vi "5785_3200MHz_multi emitter.vi"() -> ()   [LabVIEW 2021]
uses:
  <instrlib>/_niInstr/Streaming/v1/Common/Stream State.ctl
  <vilib>/Platform/TimedLoop/XDataNode/timing_clust.ctl
  <vilib>/Platform/TimedLoop/XDataNode/nitl_modes.ctl
  <vilib>/Platform/TimedLoop/XDataNode/wakeup.ctl
  <instrlib>/FlexRIO/API/FPGA/v1/Types/Start Trigger IO Resources.ctl
  <instrlib>/_niInstr/DSP/v1/Shared/Public/IQ Data.ctl
  <vilib>/rvi/Emulation/niFpgaSctlEmulationGetInTimedLoop.vi
  <vilib>/rvi/Emulation/niFpgaEmulationReportErrorSimple.vi
  <vilib>/rvi/Emulation/niFpgaGetClockAttributes.vi
  <vilib>/rvi/Emulation/niFpgaCriticalErrorInLSC.vi
  7192f61d-e408-4cca-baff-cb10c33219c0.vi
  <vilib>/rvi/interface/RandomDataEmulation/nirviRandomDataMultiElementFPGAFIFO.vi
  <instcachedir>/0/nirviRandomDataMultiElementFPGAFIFO_3E9965BA1FAD4E7B8DABA31768A09B1F.lvgen/nirviRandomDataMultiElementFPGAFIFO_3E9965BA1FAD4E7B8DABA31768A09B1F_000.vi
  <vilib>/rvi/interface/RandomDataEmulation/niFpgaRandomDataHandleErrors.vi
  <vilib>/rvi/eio/common/nirviEmuTemplateMethod_errors.vi
  <vilib>/Platform/TimedLoop/XDataNode/XDataNode.xnode
  <vilib>/rvi/DataTransferAndStorage/Container/XNode/niFpgaContainer.xnode
  <vilib>/rvi/interface/RandomDataEmulation/nirviRandomDataFpgaMultiElementTemplate.vi
  <vilib>/eio/EIONode/EIONode.xnode
  <vilib>/Platform/TimedLoop/XDataNode/XDNodeRunTimeDep.lvlib
  <instrlib>/_niInstr/Streaming/v1/FPGA/niInstr Streaming v1 FPGA.lvlib
  <instrlib>/FlexRIO/API/FPGA/v1/FlexRIO API FPGA v1.lvlib
  <instrlib>/FlexRIO/API/FPGA/v1/IO/NI5785/FlexRIO 5785 FPGA v1.lvlib
  <instrlib>/_niInstr/DSP/v1/Shared/niInstr DSP v1 Shared.lvlib
  <instrlib>/_niInstr/Basic Elements/v1/FPGA/niInstr Basic Elements v1 FPGA.lvlib
  <instrlib>/_niInstr/Streaming/v1/Common/niInstr Streaming v1 Common.lvlib
panel:
  out "pulse TX status":T1
  in  "reset system clock":bool
  in  "User-defined Start Trigger - AO":bool
  in  "flexrio.trigger.start.cfg 1":u16
  out "IO Socket\\AO Ready For Input":bool
  in  "stream.request state 1":T2
  in  "stream.num samples 1":u64
  out "stream.metadata 1":u64
  out "stream.samples transferred 1":u64
  out "stream.state 1":T2
  out "flexrio.module.io ready 0":bool
  out "flexrio.module.io error 0":i32
  out "flexrio.module.data valid 0":bool
  # "Data Path Configuration"
  # "AI Trigger Configuration"
  # "AI Stream Configuration"
  # "AO Stream Configuration"
  # "Module Status"
  # "AO Buffer Configuration"
  # "Device Utilization\n---------------------------\nTotal Slices: 62.6% (18977 out of 30300)\nSlice Registers: 23.8% (115206 out of 484800)\nSlice LUTs: 38.2% (92532 out of 242400)\nBlock RAMs: 56.8% (341 out of 600)\nDSP48s: 0.3% (6 out of 1920)\n\nNote: Utilization numbers are for the KU040. Exact values will vary for the KU060 and KU035."
  # "User-defined Controls"
  # "AO Trigger Configuration"
  # "Utilization numbers are for the KU060."
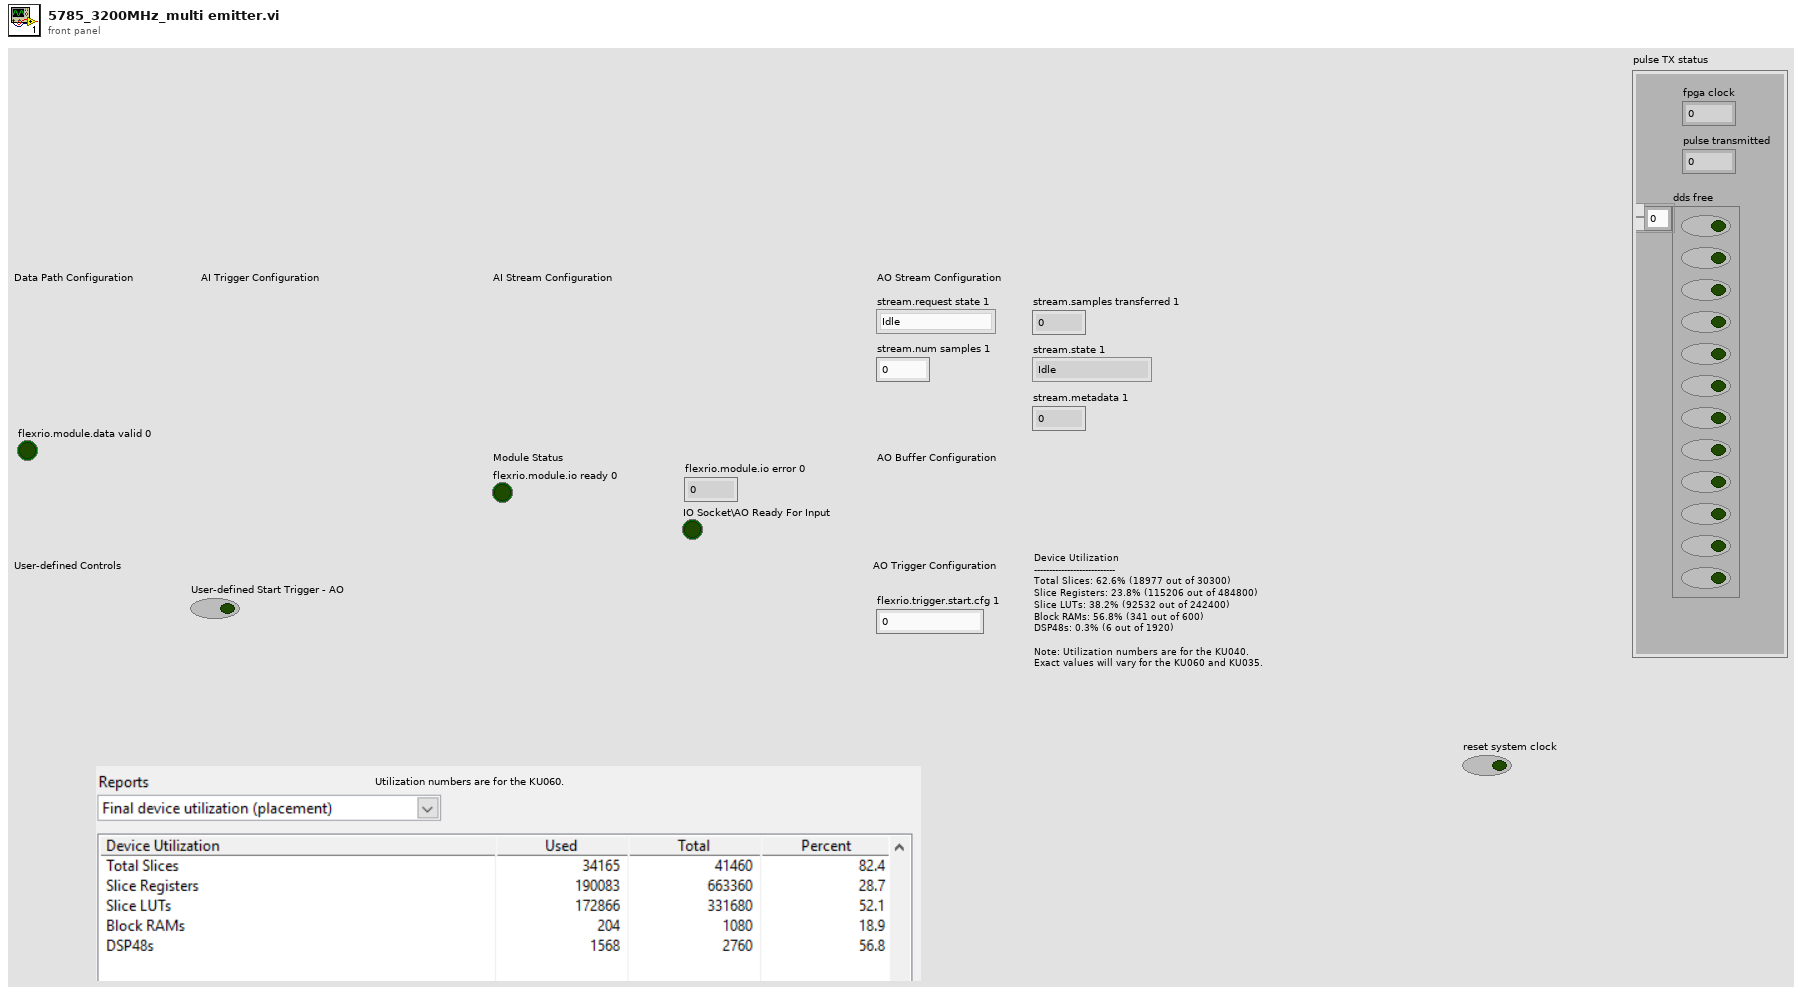
[diagram p1: front panel]
types:
  T1 = cluster{"fpga clock":u64, "pulse transmitted":u32, "dds free":bool[]}
  T2 = typedef "niInstr Streaming v1 Common.lvlib/Stream State.ctl" = enum8{"Idle", "Finite Transfer", "Continuous", "Done", "Error", "Not Ready", "Cancel"}
  T3 = typedef "XDNodeRunTimeDep.lvlib/timing_clust.ctl" = cluster{"Expected End [f-1]":u64, "Actual End [f-1]":u64, "Finished Late? [f-1]":bool, "Expected End [i-1]":u64, "Actual End [i-1]":u64, "Finished Late? [i-1]":bool, "Expected Start [i]":u64, "Actual Start [i]":u64, "Expected Start [f]":u64, "Actual Start [f]":u64, "Source Name":string, "Structure Name":string, "Period":i64, "Deadline":i64, "Offset":i64, "Start":i64, "Priority":i32, "Timeout":i32, "Mode":T4, "Wakeup Reason":T5, "Error":errorcluster, "Source Type":string, "Secondary Source Type":string, "Global End Time":u64, "Global Start Time":u64, "Frame Duration":u64, "Iteration Duration":u64, "Assigned CPU":i32, "I/O Scan Engine Mode":u32}
  T4 = typedef "XDNodeRunTimeDep.lvlib/nitl_modes.ctl" = enum32{"No Change", "Process missed periods, maintain original phase", "Discard missed periods, maintain original phase", "Process missed periods, ignore original phase", "Discard missed periods, ignore original phase"}
  T5 = typedef "XDNodeRunTimeDep.lvlib/wakeup.ctl" = enum32{"Normal", "Aborted", "Asynchronous wakeup", "Timing source error", "Timed loop error", "Timeout"}
  T6 = typedef "niInstr DSP v1 Shared.lvlib/IQ Data.ctl" = cluster{"I":fxp<+/-,18,1>, "Q":fxp<+/-,18,1>, "overflow":bool}
  T7 = typedef "FlexRIO API FPGA v1.lvlib/Start Trigger IO Resources.ctl" = cluster{"start trigger":refnum<k21>, "started event":refnum<k21>, "start trigger for export":refnum<k21>, "start trigger for tclk":refnum<k21>}
  T8 = typedef "FlexRIO API FPGA v1.lvlib/Start Trigger Control.ctl" = cluster{"arm start":bool, "done":bool}
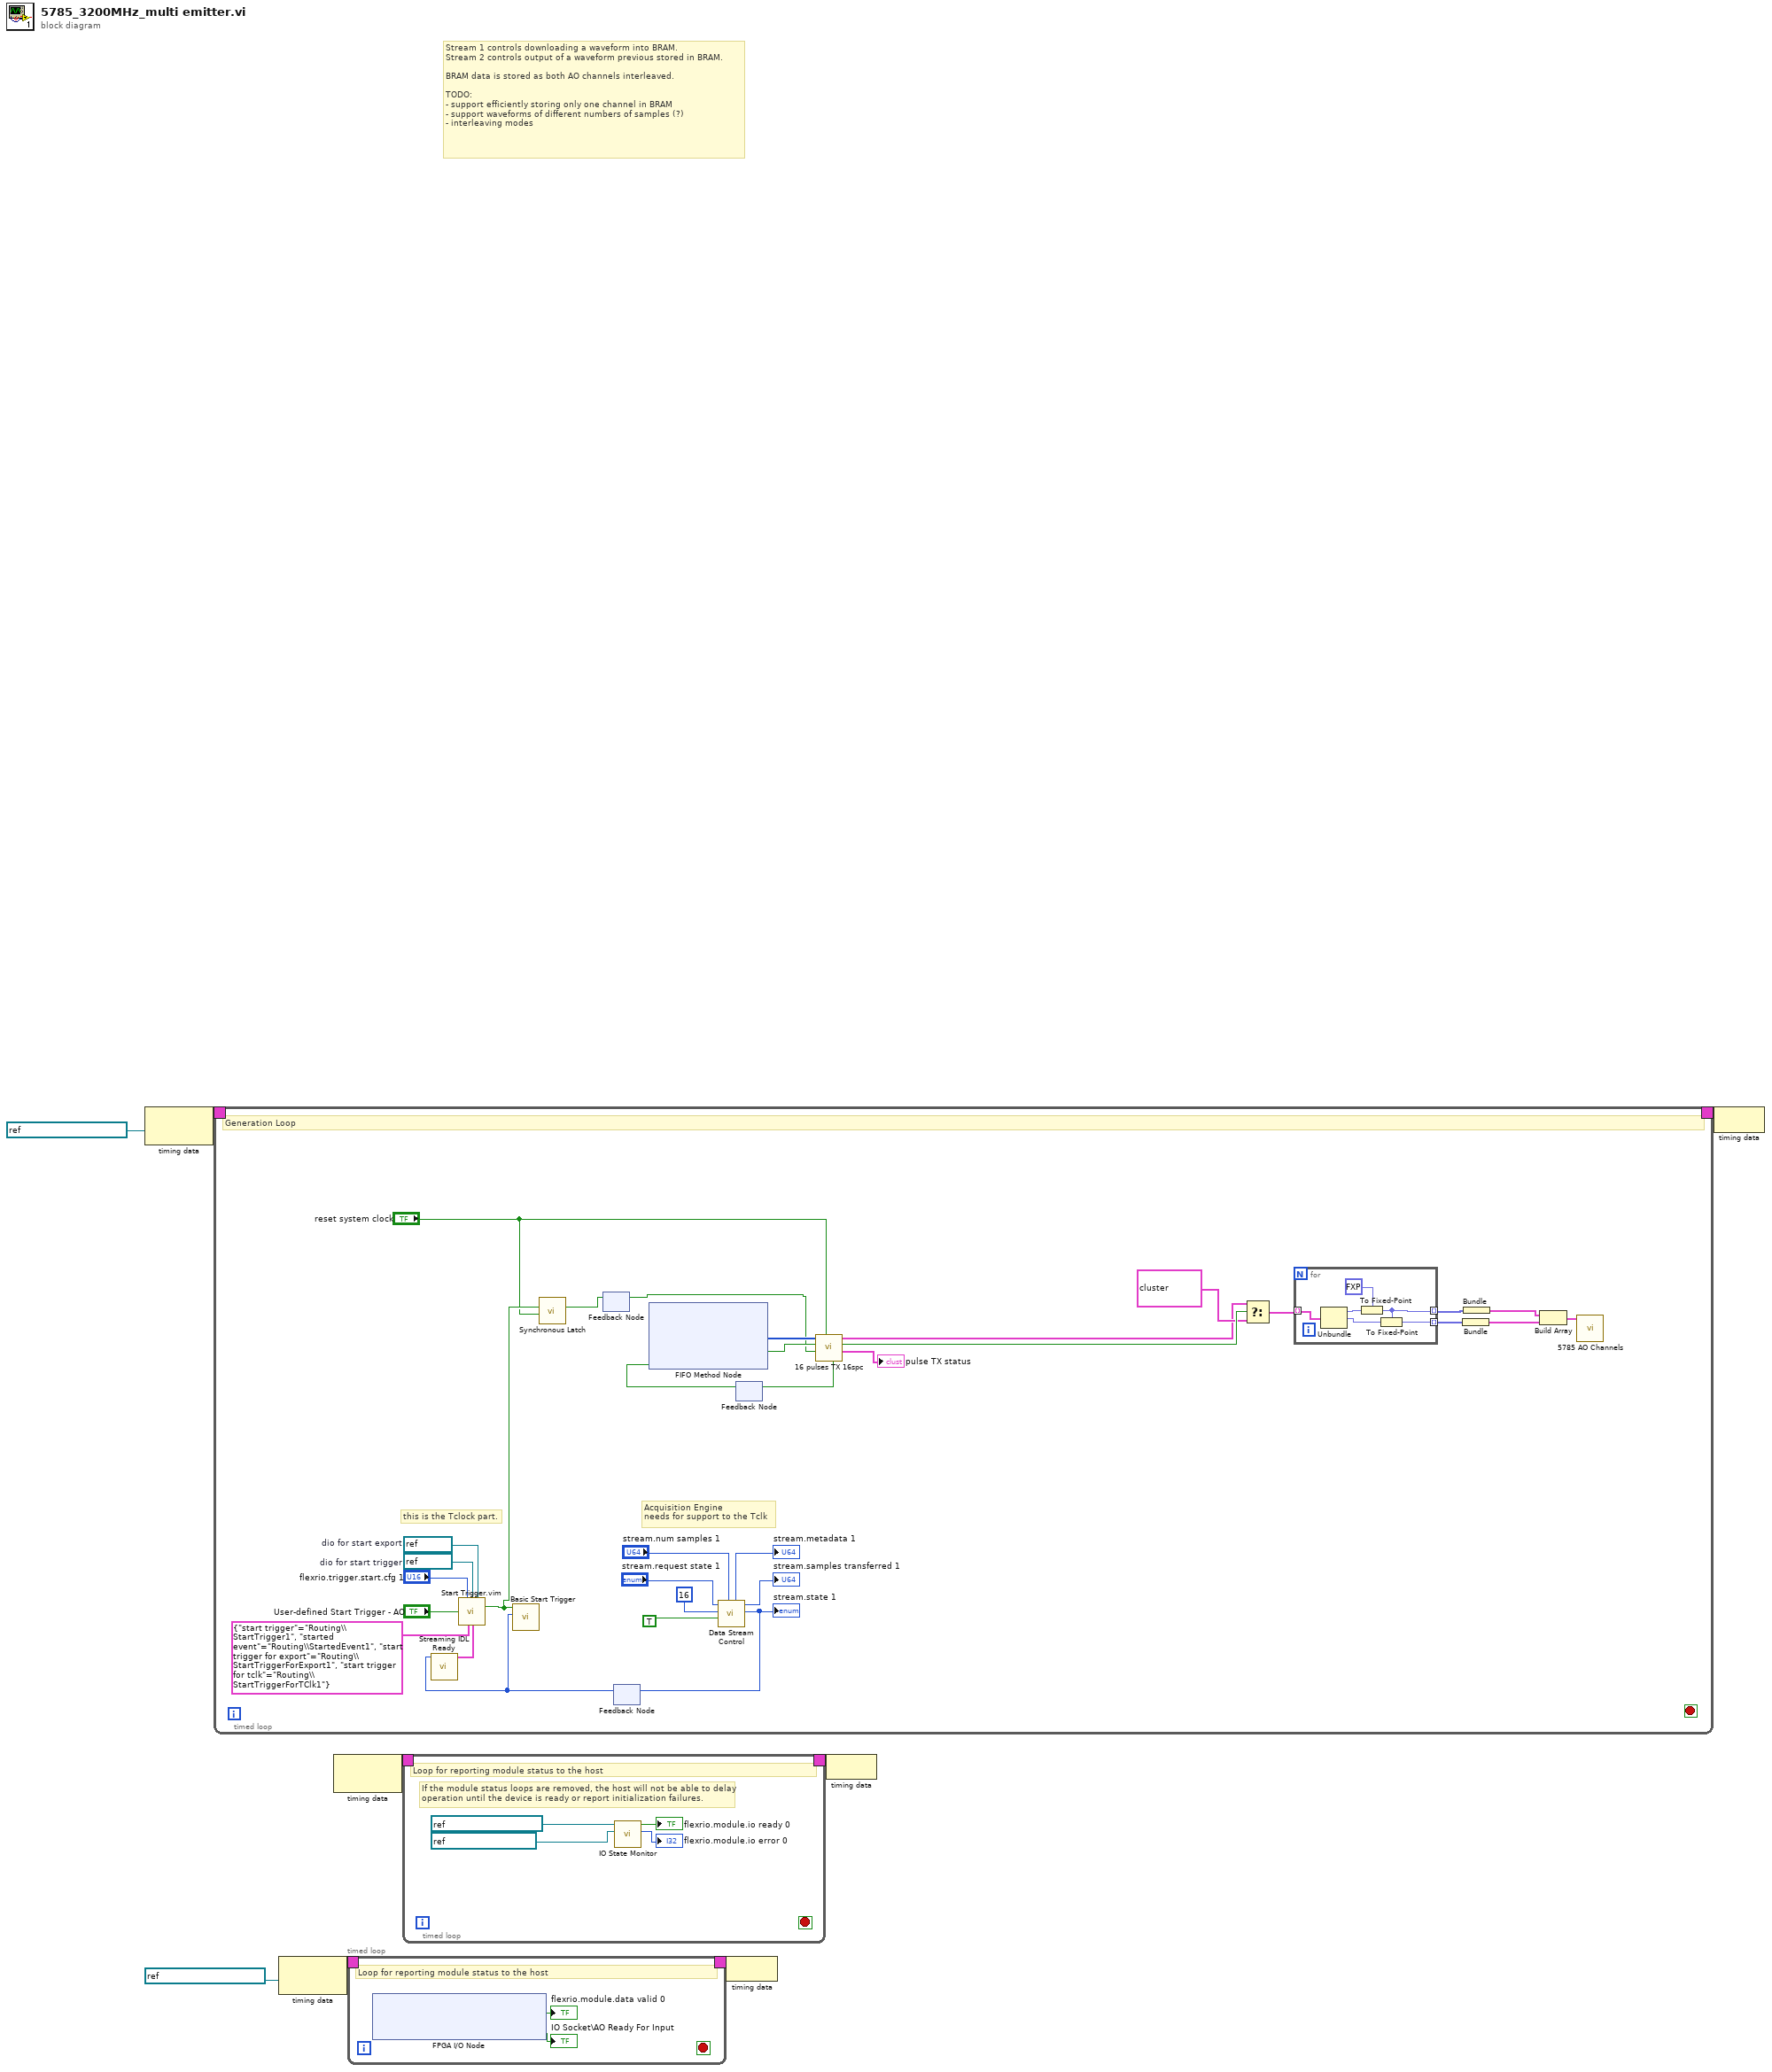
[diagram p0: block diagram]
diagram:
  # "Stream 1 controls downloading a waveform into BRAM.\nStream 2 controls output of a waveform previous stored in BRAM.\n\nBRAM data is stored as both AO channels interleaved.\n\nTODO:\n- support efficiently storing only one channel in BRAM\n- support waveforms of different numbers of samples (?)\n- interleaving modes"
  n1 = node-c288(refnum<k21> "IO Socket\\Data Clock" ("Source Name")) -> (w8:T3)
  n2 = timed-loop {
    timing: w8 -> [_]
    timing-out: [_] -> w7
    stop <- _ stop-if-true
    w30 = refnum<k21> "DIO 2"  # dio for start trigger
    w29 = refnum<k21> "DIO 3"  # dio for start export
    # "Acquisition Engine\nneeds for support to the Tclk"
    # "this is the Tclock part."
    # "Generation Loop"
    n3 = feedback #1() -> (w9:bool)  [unwired: 1 in]
    n4 = feedback #2() -> (w27:T2)  [unwired: 1 in]
    n5 = call <instrlib>:"Streaming IDL Ready.vi"("stream.state"=w27) -> ("start trigger control"=w31:T8)  [unwired: 10 in]
    n6 = call "Start Trigger.vim"("flexrio.trigger.start.cfg 0"="flexrio.trigger.start.cfg 1", "dio start"=w30, "dio for start export"=w29, "user-defined start trigger"="User-defined Start Trigger - AO", "trigger io resources"=T7 {"start trigger"="Routing\\StartTrigger1", "started event"="Routing\\StartedEvent1", "start trigger for export"="Routing\\StartTriggerForExport1", "start trigger for tclk"="Routing\\StartTriggerForTClk1"}, "start trigger control"=w31) -> ("conditioned start trigger"=w12:bool)  [unwired: 7 in, 2 out]
    n7 = call <instrlib>:"Basic Start Trigger.vi"("stream.state"=w27, "start trigger"=w12) -> ()  [unwired: 9 in, 1 out]
    n8 = call <instrlib>:"Synchronous Latch.vi"("clear"="reset system clock", "set"=w12) -> ("out"=w10:bool)  [unwired: 9 in]
    n9 = feedback-in #1(w10) -> ()
    n10 = call <instrlib>:"Data Stream Control.vi"("stream.num samples 0"="stream.num samples 1", "data valid"=TRUE, "element count"=u16 16, "stream.request state 0"="stream.request state 1") -> ("stream.state 0"=w33:T2, "stream.samples transferred 0"=→"stream.samples transferred 1":u64, "stream.metadata 0"=→"stream.metadata 1":u64)  [unwired: 3 in, 2 out]
    "stream.state 1" <- w33
    n11 = feedback-in #2(w33) -> ()
    n12 = feedback #3() -> (w24:bool)  [unwired: 1 in]
    n13 = xnode ("FIFO Method Node")("Ready for Output"=w24) -> ("Element"=w23:u64[], "Output Valid"=w22:bool)  [unwired: 1 in, 1 out]
    n14 = call "16 pulses TX 16spc.vi"("reset system clock"="reset system clock", "IQ_run"=w9, "PDW input Valid"=w22, "array PDW"=w23) -> ("pulse TX status"=→"pulse TX status":T1, "output valid"=w20:bool, "IQ out"=w18:T6[], "ready for input"=w25:bool)  [unwired: 4 in]
    n15 = feedback-in #3(w25) -> ()
    n16 = Select(t=w18, s=w20, f=T6[] [{"I"=0.0, "Q"=0.0, "overflow"=FALSE}, {"I"=0.0, "Q"=0.0, "overflow"=FALSE}, {"I"=0.0, "Q"=0.0, "overflow"=FALSE}, {"I"=0.0, "Q"=0.0, "overflow"=FALSE}, {"I"=0.0, "Q"=0.0, "overflow"=FALSE}, {"I"=0.0, "Q"=0.0, "overflow"=FALSE}, {"I"=0.0, "Q"=0.0, "overflow"=FALSE}, {"I"=0.0, "Q"=0.0, "overflow"=FALSE}, {"I"=0.0, "Q"=0.0, "overflow"=FALSE}, {"I"=0.0, "Q"=0.0, "overflow"=FALSE}, {"I"=0.0, "Q"=0.0, "overflow"=FALSE}, {"I"=0.0, "Q"=0.0, "overflow"=FALSE}, {"I"=0.0, "Q"=0.0, "overflow"=FALSE}, {"I"=0.0, "Q"=0.0, "overflow"=FALSE}, {"I"=0.0, "Q"=0.0, "overflow"=FALSE}, {"I"=0.0, "Q"=0.0, "overflow"=FALSE}]) -> (s? t:f=w17:T6[])
    n17 = for {
      tunnel: w17 -> [w46] mode=indexing
      tunnel: [w42] -> w21 mode=indexing
      tunnel: [w41] -> w16 mode=indexing
      n18 = Unbundle(w46) -> ("I"=w45:fxp<+/-,18,1>, "Q"=w43:fxp<+/-,18,1>)  [unwired: 1 out]
      n19 = To Fixed-Point(fixed-point type=fxp<+/-,12,1> 0.0 ("element"), number=w45) -> (fixed-point=w42:fxp<+/-,12,1>)
      n20 = To Fixed-Point(fixed-point type=w42, number=w43) -> (fixed-point=w41:fxp<+/-,12,1>)
    }
    n21 = Bundle(w16) -> (w14:cluster{fxp<+/-,12,1>[]})  [unwired: 1 in]
    n22 = Bundle(w21) -> (w15:cluster{fxp<+/-,12,1>[]})  [unwired: 1 in]
    n23 = Build Array(w15, w14) -> (w38:cluster{fxp<+/-,12,1>[]}[])
    n24 = call <instrlib>:"5785 AO Channels.vi"("all channels"=w38) -> ()  [unwired: 15 in]
  }
  n25 = node-c288(refnum<k21> "IO Socket\\Data Clock" ("Source Name")) -> (w3:T3)
  n26 = node-c288() -> (w5:T3)  [unwired: 1 in]
  n27 = timed-loop {
    timing: w3 -> [_]
    timing-out: [_] -> w2
    stop <- _ stop-if-true
    # "Loop for reporting module status to the host"
    n28 = xnode "FPGA I/O Node"() -> ("IO Socket\\AI Data Valid"=→"flexrio.module.data valid 0":bool, "IO Socket\\AO Ready For Input"=→"IO Socket\\AO Ready For Input":bool)  [unwired: 2 in, 2 out]
  }
  n29 = timed-loop {
    timing: w5 -> [_]
    timing-out: [_] -> w4
    stop <- _ stop-if-true
    # "If the module status loops are removed, the host will not be able to delay operation until the device is ready or report initialization failures."
    # "Loop for reporting module status to the host"
    n30 = call <instrlib>:"IO State Monitor.vi"("io error resource"=refnum<k21> "IO Socket\\IO Error" ("FPGA I/O In"), "io ready resource"=refnum<k21> "IO Socket\\IO Ready" ("FPGA I/O In")) -> ("flexrio.module.io error 0"=→"flexrio.module.io error 0":i32, "flexrio.module.io ready 0"=→"flexrio.module.io ready 0":bool)  [unwired: 8 in]
  }
  n31 = node-c288(w2) -> ()
  n32 = node-c288(w4) -> ()
  n33 = node-c288(w7) -> ()
